vi "Host - 3D display.vi"(7 "Heading":sgl, 8 "error in":errorcluster, 9 "Pitch":sgl, 10 "Roll":sgl, 11 "SceneObject in":refnum<vi>) -> (0 "error out":errorcluster, 3 "SceneObject out":refnum<vi>)   [LabVIEW 2021]
uses:
  <vilib>/picture/3D Picture Control/NI_3D Picture Control.lvlib
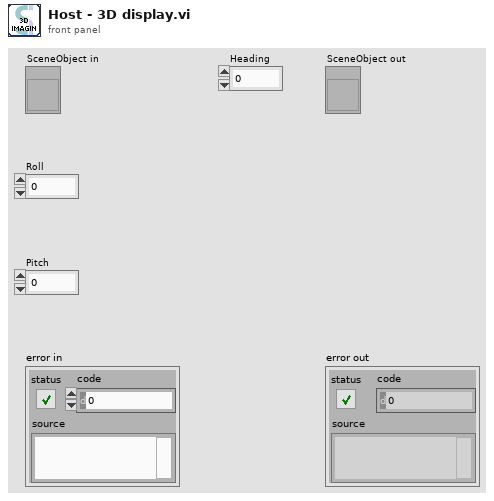
[diagram p1: front panel]
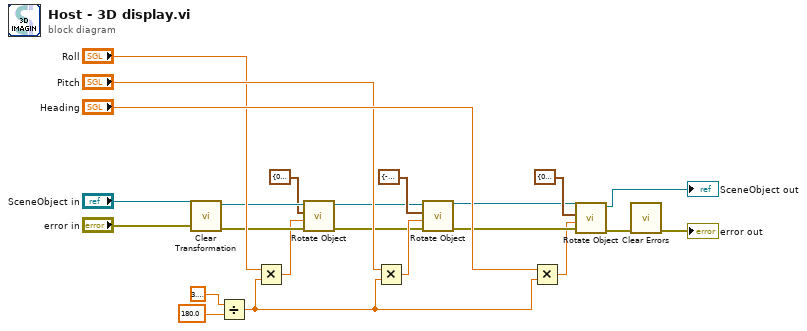
[diagram p0: block diagram]
diagram:
  n1 = call <vilib>:"Clear Transformation.vi"("error in (no error)"="error in", "Object Refnum In"="SceneObject in") -> ("error out"=w18:errorcluster, "Object Refnum Out"=w17:refnum<vi>)  [unwired: 8 in]
  n2 = Divide(x=3.141592653589793, y=180.0) -> (x/y=w23:dbl)
  n3 = Multiply(x="Roll", y=w23) -> (x*y=w11:dbl)
  n4 = call <vilib>:"Rotate Object.vi"("error in (no error)"=w18, "Angle"=w11, "Axis"=cluster{"X":sgl, "Y":sgl, "Z":sgl} {"X"=0.0, "Y"=-1.0, "Z"=0.0}, "Scene.Object In"=w17) -> ("error out"=w4:errorcluster, "Scene.Object Out"=w5:refnum<vi>)  [unwired: 6 in]
  n5 = Multiply(x="Pitch", y=w23) -> (x*y=w12:dbl)
  n6 = call <vilib>:"Rotate Object.vi"("error in (no error)"=w4, "Angle"=w12, "Axis"=cluster{"X":sgl, "Y":sgl, "Z":sgl} {"X"=-1.0, "Y"=0.0, "Z"=0.0}, "Scene.Object In"=w5) -> ("error out"=w19:errorcluster, "Scene.Object Out"=w3:refnum<vi>)  [unwired: 6 in]
  n7 = Multiply(x="Heading", y=w23) -> (x*y=w13:dbl)
  n8 = call <vilib>:"Rotate Object.vi"("error in (no error)"=w19, "Angle"=w13, "Axis"=cluster{"X":sgl, "Y":sgl, "Z":sgl} {"X"=0.0, "Y"=0.0, "Z"=-1.0}, "Scene.Object In"=w3) -> ("error out"=w2:errorcluster, "Scene.Object Out"=→"SceneObject out":refnum<vi>)  [unwired: 6 in]
  n9 = call <vilib>:"Clear Errors.vi"("error in (no error)"=w2) -> ("error out"=→"error out":errorcluster)  [unwired: 5 in, 1 out]
